vi "Set JSON Data.vi"(7 "VI Reference":refnum<vi>, 8 "error in (no error)":errorcluster, 10 "Value":string, 11 "Boolean In":refnum<class "Boolean.lvclass">) -> (0 "error out":errorcluster, 3 "Boolean Out":refnum<class "Boolean.lvclass">)   [LabVIEW 2017, in "Front Panel Publisher.lvlib" / "Boolean.lvclass"]
uses:
  Boolean.lvclass
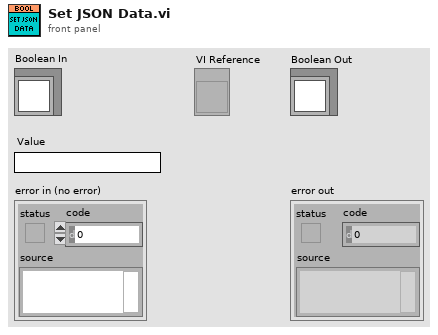
[diagram p1: front panel]
types:
  T1 = typedef "Front Panel Publisher.lvlib/Boolean.lvclass/Attributes.ctl" = cluster{"Boolean ref":refnum<vi>, "Switching":bool, "Boolean Strings":string[], "Text":refnum<class "Text.lvclass">, "Images b64":string[]}
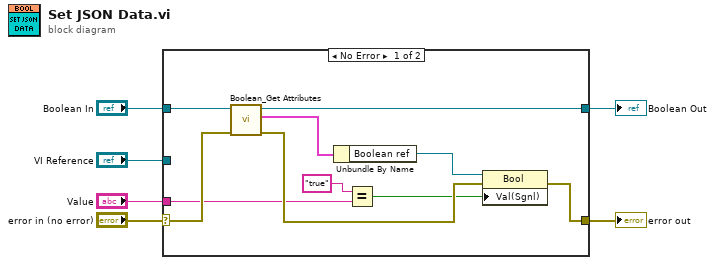
[diagram p0: block diagram]
diagram:
  n1 = case shown="No Error" "error in (no error)" {
    selector: "error in (no error)" -> [w16 w18]
    tunnel: [w15 w18] -> w5
    tunnel: [w11 w17] -> w3
    tunnel: "Boolean In" -> [w12 w17]
    tunnel: "Value" -> [w10 _]
    tunnel: "VI Reference" -> [_ _]
    frame No Error {
      n2 = call "Boolean_Get Attributes.vi"("error in (no error)"=w16, "Boolean In"=w12) -> ("error out"=w14:errorcluster, "Boolean Attributes"=w13:T1, "Boolean Out"=w11:refnum<class "Boolean.lvclass">)  [unwired: 7 in]
      n3 = Unbundle By Name(w13) -> ("Boolean ref"=w7:refnum<vi>)
      n4 = Equal?(x="true" ("y"), y=w10) -> (x = y?=w8:bool)
      n5 = property class="Bool"(reference=w7, error in=w14, "Val(Sgnl)"=w8) -> (error out=w15:errorcluster)  [unwired: 1 out]
    }
    frame Error {
    }
  }
  "error out" <- w5
  "Boolean Out" <- w3
